vi "MS debouncer FGV.vi"(1 "Iterations":i32=10, 2 "At target?":bool=TRUE) -> (0 "Is stabe":bool)   [LabVIEW 2022 SP3, in "Magnet module.lvlib"]
doc: "This is special FGV. It should be called every second. If magnet is on target more than given number of iteration, field is considered as stable."
uses:
  Magnet module.lvlib
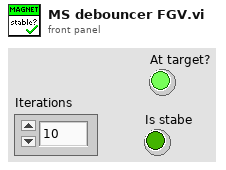
[diagram p1: front panel]
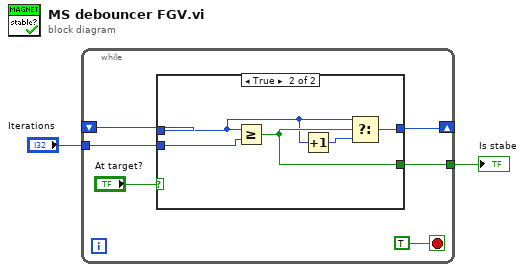
[diagram p0: block diagram]
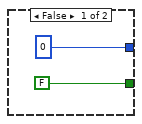
[diagram p2: hidden frame]
diagram:
  n1 = while {
    shift-right: [w5] -> _
    shift-left: _ -> [w7]
    tunnel: [w6] -> w2
    tunnel: "Iterations" -> [w3]
    stop <- TRUE stop-if-true
    n2 = case shown="True" "At target?" {
      tunnel: w7 -> [_ w13]
      tunnel: [FALSE w15] -> w6
      tunnel: [0 ("Numeric Control") w12] -> w5
      tunnel: w3 -> [_ w11]
      frame False {
      }
      frame True {
        n3 = Greater Or Equal?(x=w13, y=w11) -> (x >= y?=w15:bool)
        n4 = Increment(x=w13) -> (x+1=w14:i32)
        n5 = Select(t=w13, s=w15, f=w14) -> (s? t:f=w12:i32)
      }
    }
  }
  "Is stabe" <- w2
